vi "Set_Acceleration.vi"(8 "error in (no error)":errorcluster, 10 "Set_ACC":i32, 11 "connection ID":refnum<k5>) -> (0 "error out":errorcluster, 3 "TCP Network Connection out":refnum<k5>)   [LabVIEW 2019]
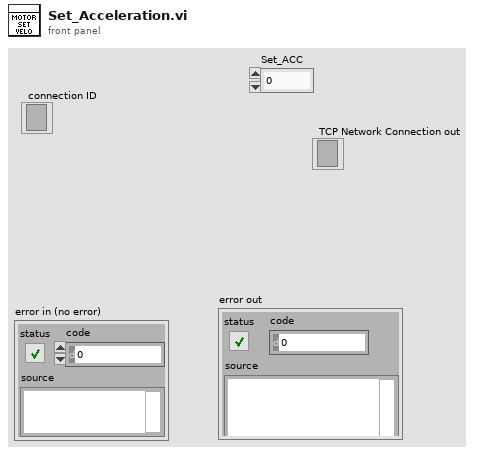
[diagram p1: front panel]
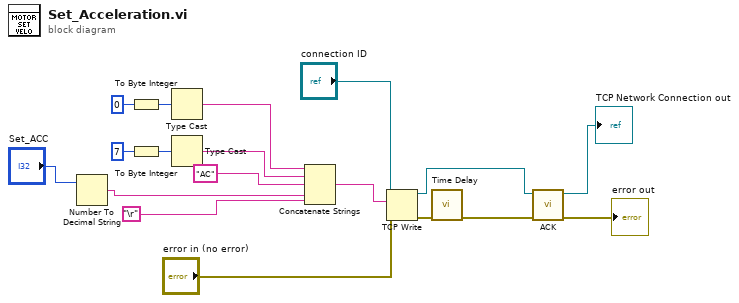
[diagram p0: block diagram]
diagram:
  n1 = Number To Decimal String(number="Set_ACC") -> (decimal integer string=w2:string)  [unwired: 1 in]
  n2 = To Byte Integer(number=i8 0) -> (8bit integer=w13:i8)
  n3 = To Byte Integer(number=i8 7) -> (8bit integer=w16:i8)
  n4 = Type Cast(x=w13) -> (*(type *) &x=w14:string)  [unwired: 1 in]
  n5 = Type Cast(x=w16) -> (*(type *) &x=w15:string)  [unwired: 1 in]
  n6 = Concatenate Strings(w14, w15, "AC" ("string"), w2, "\r") -> (w10:string)
  n7 = TCP Write(connection ID="connection ID", data in=w10, error in (no error)="error in (no error)") -> (connection ID out=w9:refnum<k5>, error out=w8:errorcluster)  [unwired: 1 in, 1 out]
  n8 = call "Time Delay"("error in (no error)"=w8) -> ("error out"=w7:errorcluster)  [unwired: 10 in]
  n9 = call "ACK.vi"("error in (no error)"=w7, "TCP Network Connection in"=w9) -> ("error out"=→"error out":errorcluster, "TCP Network Connection out"=→"TCP Network Connection out":refnum<k5>)  [unwired: 7 in, 1 out]
